vi "Feeding_SCAN_CHECK.vi"(7 "CYCLE DATA IN":T1, 8 "error in (no error)":errorcluster, 11 "raw scan code":string) -> (0 "error out":errorcluster, 5 "CYCLE DATA OUT":T1)   [LabVIEW 2017]
uses:
  Controls/Feed_Cyc_Data.ctl
  Controls/QUEUE_STATES.ctl
  Controls/Feed_St.ctl
  <vilib>/Utility/file.llb/Read Delimited Spreadsheet (string).vi
  <vilib>/Utility/file.llb/Write Delimited Spreadsheet (string).vi
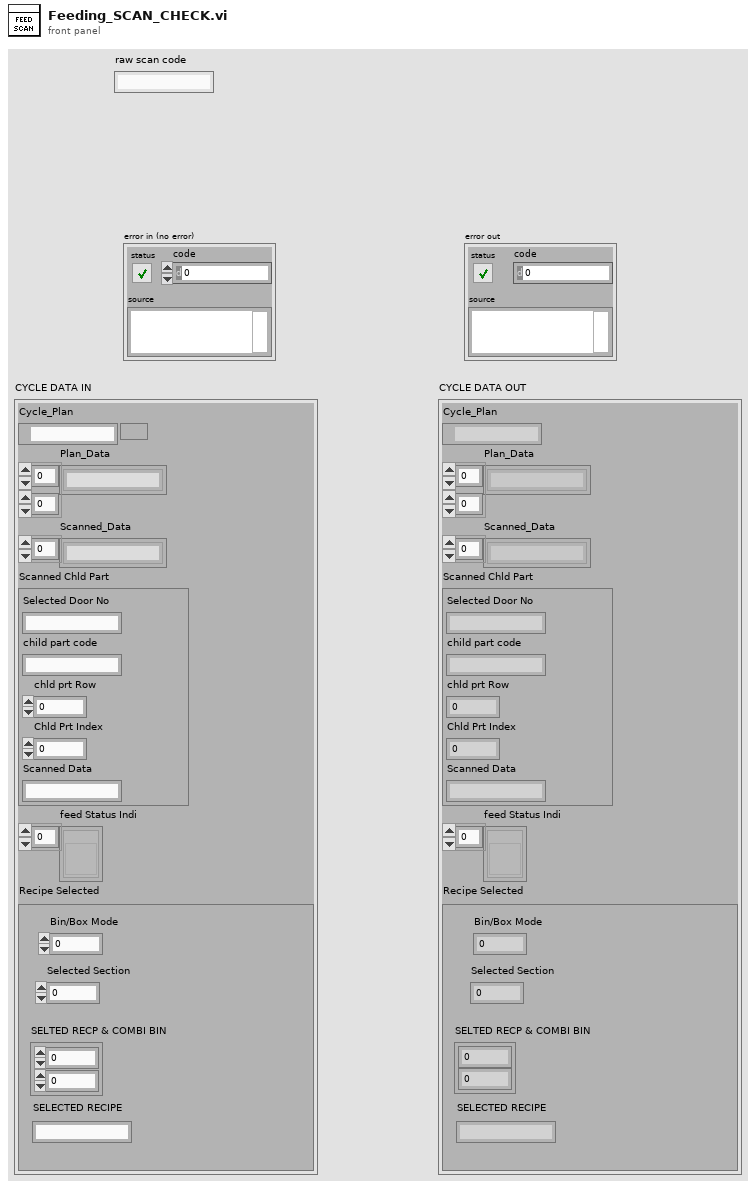
[diagram p1: front panel]
types:
  T1 = typedef "Feed_Cyc_Data.ctl" = cluster{"Cycle_Plan":path, "Plan_Data":string[][], "Scanned_Data":string[], "Scanned Chld Part":cluster{"Selected Door No":string, "child part code":string, "chld prt Row":i32, "Chld Prt Index":i32, "Scanned Data":string}, "feed Status Indi":refnum<vi>[], "Recipe Selected":cluster{"Bin/Box Mode":i32, "Selected Section":i32, "SELTED RECP & COMBI BIN":cluster{i32, i32}, "SELECTED RECIPE":string}}
  T2 = typedef "Feed_St.ctl" = enum16{"Int 2", "Cluster_update", "Read_Plan", "QR_Scanned", "Int", "SaveReport ", "Error_Handler", "Wait", "Close_Door", "Stop"}
  T3 = typedef "QUEUE_STATES.ctl" = enum16{"CREATE Q", "EN Q", "DE Q", "CLOSE Q"}
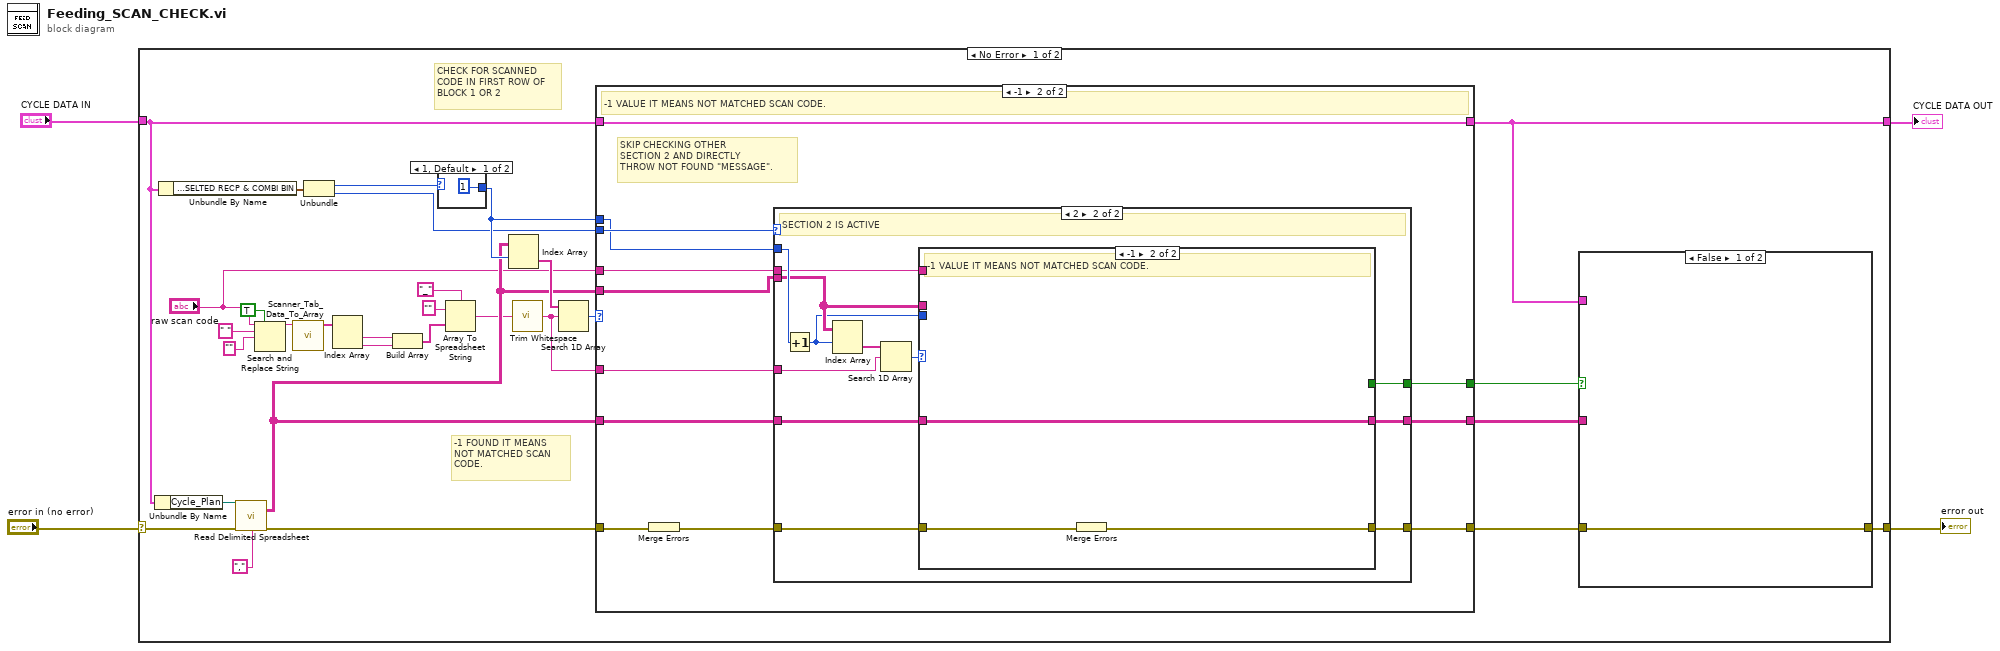
[diagram p0: block diagram]
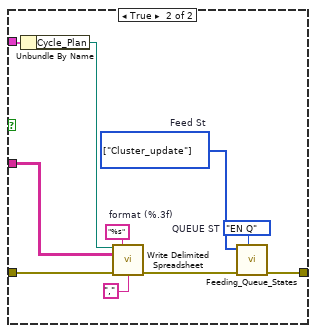
[diagram p2: hidden frame]
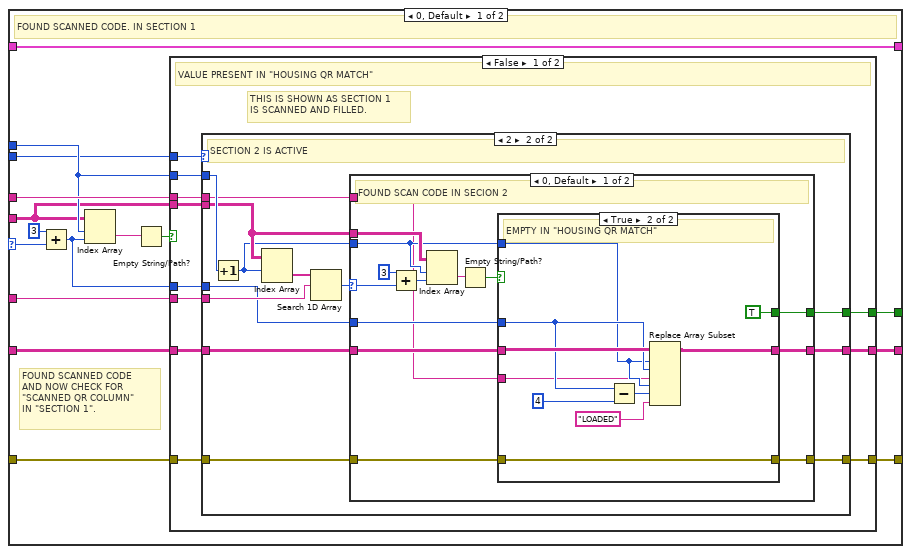
[diagram p3: hidden frame]
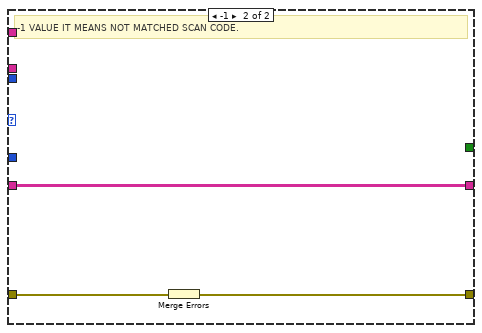
[diagram p6: hidden frame]
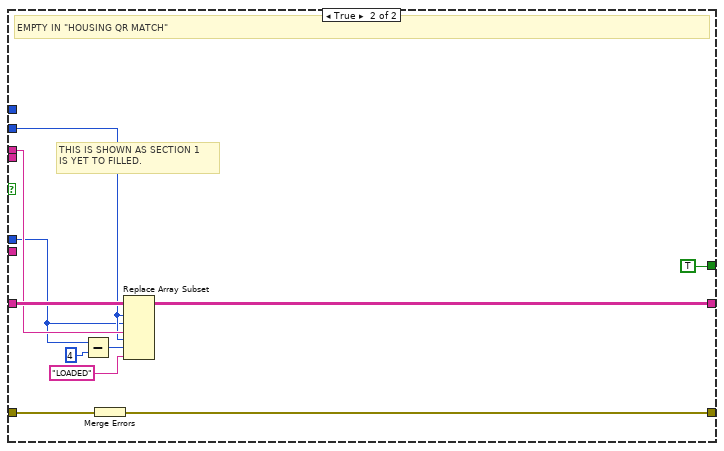
[diagram p7: hidden frame]
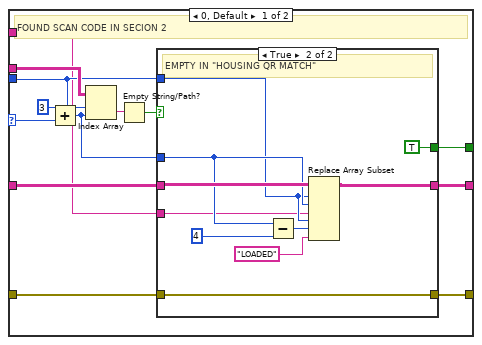
[diagram p9: hidden frame]
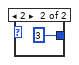
[diagram p11: hidden frame]
diagram:
  n1 = case shown="No Error" "error in (no error)" {
    selector: "error in (no error)" -> [w31 w185]
    tunnel: [w15 w185] -> w3
    tunnel: [w13 w184] -> w1
    tunnel: "CYCLE DATA IN" -> [w20 w184]
    frame No Error {
      # "-1 FOUND IT MEANS\nNOT MATCHED SCAN\nCODE."
      # "CHECK FOR SCANNED\nCODE IN FIRST ROW OF\nBLOCK 1 OR 2"
      n2 = Unbundle By Name(w20) -> ("Cycle_Plan"=w32:path)
      n3 = Unbundle By Name(w20) -> ("Recipe Selected.SELTED RECP & COMBI BIN"=w29:cluster{i32, i32})
      n4 = call-poly <vilib>:"Read Delimited Spreadsheet.vi"("file path (dialog if empty)"=w32, "error in (no error)"=w31, "delimiter (\\t)"=",") -> ("all rows"=w17:string[][], "error out"=w30:errorcluster)  [unwired: 7 in, 4 out]
      n5 = Search and Replace String(replace all?=TRUE, input string="raw scan code", search string=" ", replace string="") -> (result string=w27:string)  [unwired: 4 in, 3 out]
      n6 = call "Scanner_Tab_Data_To_Array.vi"("Scanner Data"=w27) -> ("Array"=w11:string[])  [unwired: 10 in]
      n7 = Unbundle(w29) -> (w28:i32, w16:i32)
      n8 = Index Array(array=w11) -> (element #1=w10:string, element #2=w9:string)  [unwired: 2 in]
      n9 = Build Array(w10, w9) -> (w8:string[])
      n10 = case shown="1, Default" w28 {
        tunnel: [1 3] -> w18
        frame 1, Default {
        }
        frame 2 {
        }
      }
      n11 = Array To Spreadsheet String(delimiter (Tab)="_", array=w8, 3:"") -> (spreadsheet string=w7:string)
      n12 = Index Array(array=w17, index (row)=w18) -> (element=w21:string[])  [unwired: 1 in]
      n13 = call <vilib>:"Trim Whitespace.vi"("string"=w7) -> ("trimmed string"=w5:string)  [unwired: 1 in]
      n14 = Search 1D Array(1D array=w21, element=w5) -> (index of element=w19:i32)  [unwired: 1 in]
      n15 = case shown="-1" w19 {
        selector: w19 -> [w60 _]
        tunnel: [w57 w130] -> w34
        tunnel: w30 -> [w61 w139]
        tunnel: [w54 w138] -> w13
        tunnel: w20 -> [w54 w138]
        tunnel: w17 -> [w48 w135]
        tunnel: w18 -> [w52 w129]
        tunnel: "raw scan code" -> [w55 w136]
        tunnel: w17 -> [w53 w134]
        tunnel: [w50 w133] -> w12
        tunnel: w16 -> [w49 w137]
        tunnel: w5 -> [w47 w128]
        tunnel: [w46 w132] -> w14
        frame 0, Default {
          # "FOUND SCANNED CODE\nAND NOW CHECK FOR\n\"SCANNED QR COLUMN\"\nIN \"SECTION 1\"."
          # "FOUND SCANNED CODE. IN SECTION 1"
          n16 = Add(x=3, y=w60) -> (x+y=w51:i32)
          n17 = Index Array(array=w48, index (row)=w52, index (col)=w51) -> (element=w58:string)
          n18 = Empty String/Path?(string/path=w58) -> (empty?=w56:bool)
          n19 = case shown="False" w56 {
            tunnel: w61 -> [w71 w127]
            tunnel: [w72 w126] -> w57
            tunnel: w55 -> [w63 w124]
            tunnel: w53 -> [w68 w125]
            tunnel: w52 -> [w67 w121]
            tunnel: w51 -> [w65 w120]
            tunnel: [w69 w123] -> w50
            tunnel: w49 -> [w70 _]
            tunnel: w48 -> [w66 _]
            tunnel: w47 -> [w64 _]
            tunnel: [w62 TRUE] -> w46
            frame False {
              # "THIS IS SHOWN AS SECTION 1\nIS SCANNED AND FILLED."
              # "VALUE PRESENT IN \"HOUSING QR MATCH\""
              n20 = case shown="2" w70 {
                tunnel: [w74 w83] -> w72
                tunnel: w71 -> [w74 w87]
                tunnel: [w73 w82] -> w69
                tunnel: w68 -> [w73 w81]
                tunnel: w67 -> [_ w86]
                tunnel: w66 -> [_ w79]
                tunnel: w65 -> [_ w77]
                tunnel: w64 -> [_ w84]
                tunnel: w63 -> [_ w76]
                tunnel: [_ w75] -> w62
                frame 1, Default {
                  # "ONLY SECTION 1"
                }
                frame 2 {
                  # "SECTION 2 IS ACTIVE"
                  n21 = Increment(x=w86) -> (x+1=w78:i32)
                  n22 = Index Array(array=w79, index (row)=w78) -> (element=w85:string[])  [unwired: 1 in]
                  n23 = Search 1D Array(1D array=w85, element=w84) -> (index of element=w80:i32)  [unwired: 1 in]
                  n24 = case shown="0, Default" w80 {
                    selector: w80 -> [w98 _]
                    tunnel: w87 -> [w101 w116]
                    tunnel: [w96 w115] -> w83
                    tunnel: [w93 w114] -> w82
                    tunnel: w81 -> [w92 w114]
                    tunnel: w79 -> [w97 _]
                    tunnel: w78 -> [w91 _]
                    tunnel: w77 -> [w90 _]
                    tunnel: w76 -> [w89 _]
                    tunnel: [w88 _] -> w75
                    frame 0, Default {
                      # "FOUND SCAN CODE IN SECION 2"
                      n25 = Add(x=3, y=w98) -> (x+y=w100:i32)
                      n26 = Index Array(array=w97, index (row)=w91, index (col)=w100) -> (element=w95:string)
                      n27 = Empty String/Path?(string/path=w95) -> (empty?=w94:bool)
                      n28 = case shown="True" w94 {
                        tunnel: w101 -> [w102 w113]
                        tunnel: [w102 w113] -> w96
                        tunnel: [w103 w109] -> w93
                        tunnel: w92 -> [w103 w108]
                        tunnel: w91 -> [_ w106]
                        tunnel: w90 -> [_ w107]
                        tunnel: w89 -> [_ w105]
                        tunnel: [_ TRUE] -> w88
                        frame False {
                          # "VALUE PRESENT IN \"HOUSING QR MATCH\""
                        }
                        frame True {
                          # "EMPTY IN \"HOUSING QR MATCH\""
                          n29 = Subtract(x=w107, y=4) -> (x-y=w112:i32)
                          n30 = Replace Array Subset(array=w108, new element #1=w105, index (row) #1=w106, index (col) #1=w107, new element #2="LOADED", index (row) #2=w106, index (col) #2=w112) -> (w109:string[][])
                        }
                      }
                    }
                    frame -1 {
                      # "-1 VALUE IT MEANS NOT MATCHED SCAN CODE."
                      n31 = Merge Errors(w116) -> (w115:errorcluster)
                    }
                  }
                }
              }
            }
            frame True {
              # "THIS IS SHOWN AS SECTION 1\nIS YET TO FILLED."
              # "EMPTY IN \"HOUSING QR MATCH\""
              n32 = Subtract(x=w120, y=4) -> (x-y=w122:i32)
              n33 = Merge Errors(w127) -> (w126:errorcluster)
              n34 = Replace Array Subset(array=w125, new element #1=w124, index (row) #1=w121, index (col) #1=w120, new element #2="LOADED", index (row) #2=w121, index (col) #2=w122) -> (w123:string[][])
            }
          }
        }
        frame -1 {
          # "SKIP CHECKING OTHER \nSECTION 2 AND DIRECTLY\nTHROW NOT FOUND \"MESSAGE\"."
          # "-1 VALUE IT MEANS NOT MATCHED SCAN CODE."
          n35 = Merge Errors(w139) -> (w131:errorcluster)
          n36 = case shown="2" w137 {
            tunnel: [w141 w149] -> w130
            tunnel: w131 -> [w141 w153]
            tunnel: [w140 w148] -> w133
            tunnel: w134 -> [w140 w147]
            tunnel: w129 -> [_ w152]
            tunnel: w135 -> [_ w145]
            tunnel: w128 -> [_ w150]
            tunnel: w136 -> [_ w143]
            tunnel: [_ w142] -> w132
            frame 1, Default {
              # "ONLY SECTION 1"
            }
            frame 2 {
              # "SECTION 2 IS ACTIVE"
              n37 = Increment(x=w152) -> (x+1=w144:i32)
              n38 = Index Array(array=w145, index (row)=w144) -> (element=w151:string[])  [unwired: 1 in]
              n39 = Search 1D Array(1D array=w151, element=w150) -> (index of element=w146:i32)  [unwired: 1 in]
              n40 = case shown="-1" w146 {
                selector: w146 -> [w164 _]
                tunnel: w153 -> [w166 w181]
                tunnel: [w162 w180] -> w149
                tunnel: [w159 w179] -> w148
                tunnel: w147 -> [w158 w179]
                tunnel: w145 -> [w163 _]
                tunnel: w144 -> [w157 _]
                tunnel: w143 -> [w156 _]
                tunnel: [w155 _] -> w142
                frame 0, Default {
                  # "FOUND SCAN CODE IN SECION 2"
                  n41 = Add(x=3, y=w164) -> (x+y=w154:i32)
                  n42 = Index Array(array=w163, index (row)=w157, index (col)=w154) -> (element=w161:string)
                  n43 = Empty String/Path?(string/path=w161) -> (empty?=w160:bool)
                  n44 = case shown="True" w160 {
                    tunnel: w166 -> [w167 w178]
                    tunnel: [w167 w178] -> w162
                    tunnel: [w168 w174] -> w159
                    tunnel: w158 -> [w168 w173]
                    tunnel: w157 -> [_ w171]
                    tunnel: w154 -> [_ w172]
                    tunnel: w156 -> [_ w170]
                    tunnel: [_ TRUE] -> w155
                    frame False {
                      # "VALUE PRESENT IN \"HOUSING QR MATCH\""
                    }
                    frame True {
                      # "EMPTY IN \"HOUSING QR MATCH\""
                      n45 = Subtract(x=w172, y=4) -> (x-y=w177:i32)
                      n46 = Replace Array Subset(array=w173, new element #1=w170, index (row) #1=w171, index (col) #1=w172, new element #2="LOADED", index (row) #2=w171, index (col) #2=w177) -> (w174:string[][])
                    }
                  }
                }
                frame -1 {
                  # "-1 VALUE IT MEANS NOT MATCHED SCAN CODE."
                  n47 = Merge Errors(w181) -> (w180:errorcluster)
                }
              }
            }
          }
        }
      }
      n48 = case shown="False" w14 {
        tunnel: w34 -> [w35 w44]
        tunnel: [w35 w37] -> w15
        tunnel: w13 -> [_ w43]
        tunnel: w12 -> [_ w40]
        frame False {
        }
        frame True {
          w36 = T2[] [enum."Cluster_update"] items=["Int 2", "Cluster_update", "Read_Plan", "QR_Scanned", "Int", "SaveReport ", "Error_Handler", "Wait", "Close_Door", "Stop"]  # Feed St
          w39 = QUEUE_STATES."EN Q"  # QUEUE ST
          w41 = "%s"  # format (%.3f)
          n49 = Unbundle By Name(w43) -> ("Cycle_Plan"=w42:path)
          n50 = call-poly <vilib>:"Write Delimited Spreadsheet.vi"("file path (dialog if empty)"=w42, "format (%s)"=w41, "2D data"=w40, "error in (no error)"=w44, "delimiter (\\t)"=",") -> ("error out"=w38:errorcluster)  [unwired: 9 in, 1 out]
          n51 = call "Feeding_Queue_States.vi"("QUEUE ST"=w39, "error in"=w38, "Feed St"=w36) -> ("error OUT"=w37:errorcluster)  [unwired: 7 in, 1 out]
        }
      }
    }
    frame Error {
    }
  }
  "error out" <- w3
  "CYCLE DATA OUT" <- w1
